vi "探头窗口-8-网络版.vi"() -> ()   [LabVIEW 2017]
panel:
  in  "外部停止命令？":bool=TRUE
  out "引用-监测模式？":refnum<vi>
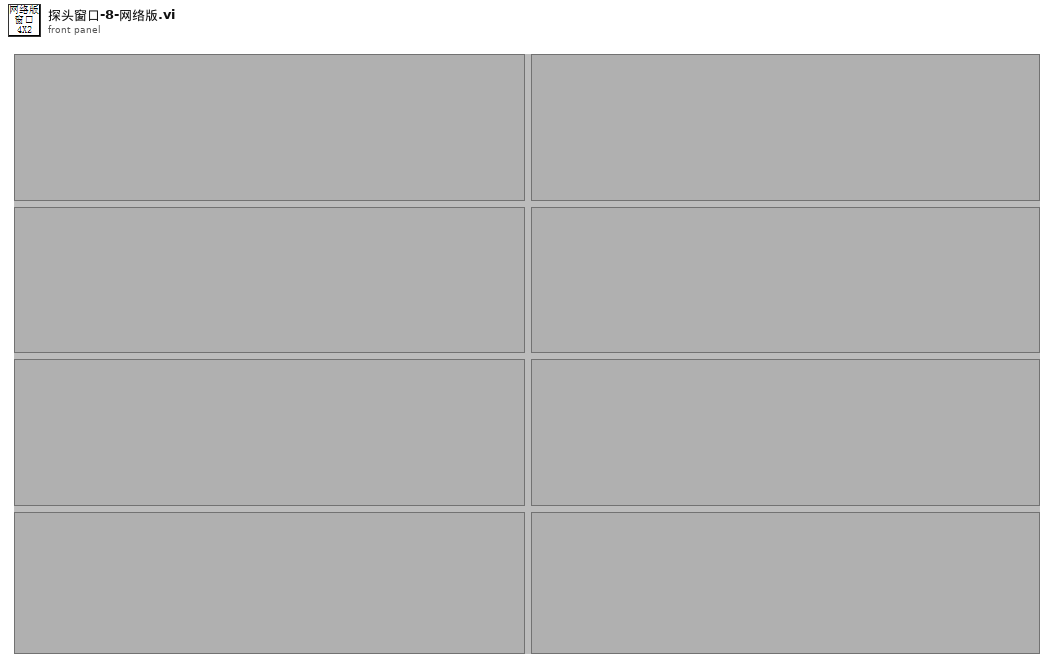
[diagram p1: front panel]
types:
  T1 = typedef "探头属性.ctl" = cluster{"探头地址与信息":T2, "测量值":T5, "限值":T6, "探头状态":T7, "累积记录":T8, "报警方式":T9}
  T2 = typedef "探测器信息.ctl" = cluster{"网络地址":string, "名称":string, "备注":string, "累积剂量":dbl, "累积限值":dbl, "硬件剂量率限值":T3, "剂量率限值1":dbl, "剂量率限值2":dbl, "报警方式":T4}
  T3 = typedef "探头剂量率限值选择.ctl" = enum16{"一级限值", "二级限值"}
  T4 = typedef "报警方式选择.ctl" = enum16{"常报警", "自动静音", "手动静音"}
  T5 = typedef "测量值.ctl" = cluster{"时间":timestamp, "数值":dbl}
  T6 = typedef "剂量率限值.ctl" = cluster{"限值1":dbl, "限值2":dbl, "探头限值":T3}
  T7 = typedef "探头状态.ctl" = enum16{"正常", "离线", "禁用", "一级报警", "二级报警", "累积报警"}
  T8 = typedef "单条累积记录.ctl" = cluster{"起始时间":timestamp, "结束时间":timestamp, "累积剂量":dbl}
  T9 = typedef "报警方式.ctl" = cluster{"报警方式":T4, "延迟计时":u16, "报警中？":bool}
  T10 = typedef "eventvkey.ctl" = enum16{"ASCII", "Enter", "Return", "Shift", "Ctrl", "Alt", "Cmd", "Opt", "Caps", "NumLock", "Clear", "Break", "Up", "Down", "Left", "Right", "Insert", "Delete", "Home", "End", "PageUp", "PageDown", "Escape", "Help", "Pause", "ScrollLock", "F1", "F2", "F3", "F4", "F5", "F6", "F7", "F8", "F9", "F10", "F11", "F12", "F13", "F14", "F15", "F16", "F17", "F18", "F19", "F20", "F21", "F22", "F23", "F24", "Play", "VolumeUp", "VolumeDown", "Mute", "Two Byte Char"}
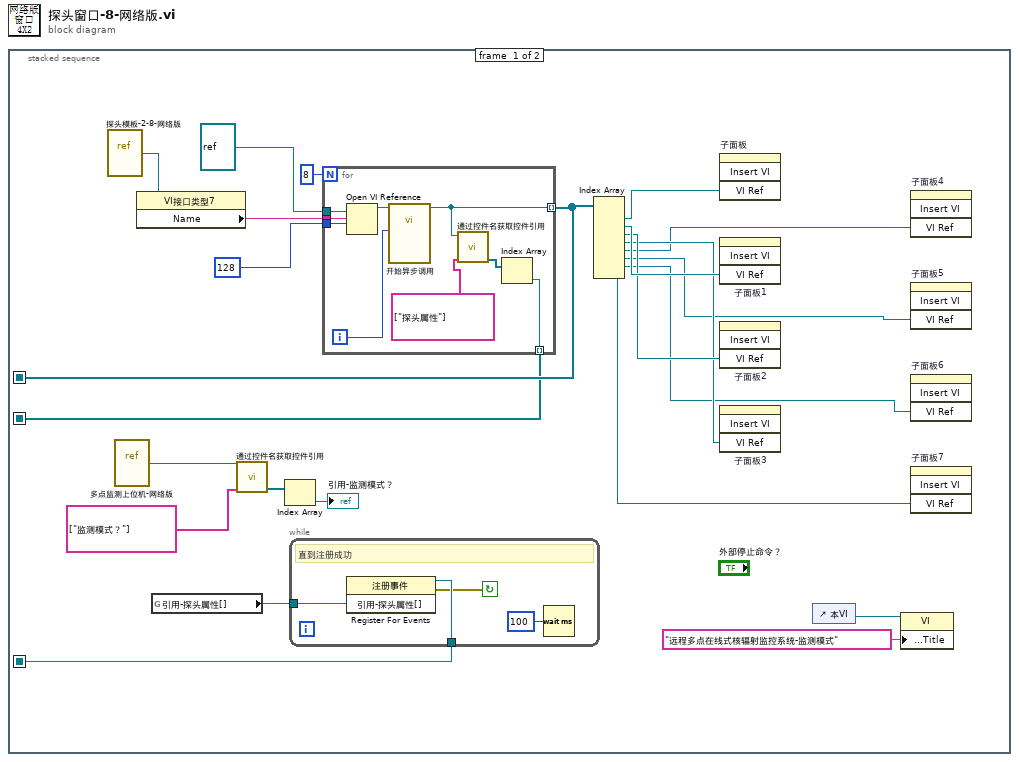
[diagram p0: block diagram]
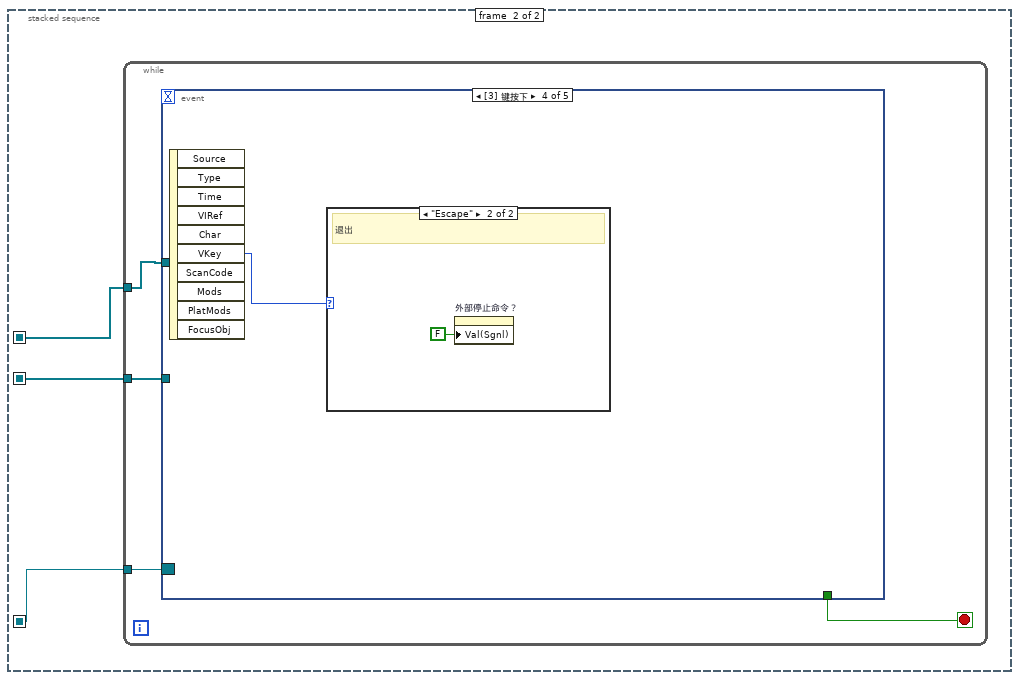
[diagram p2: hidden frame]
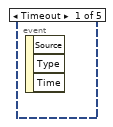
[diagram p3: hidden frame]
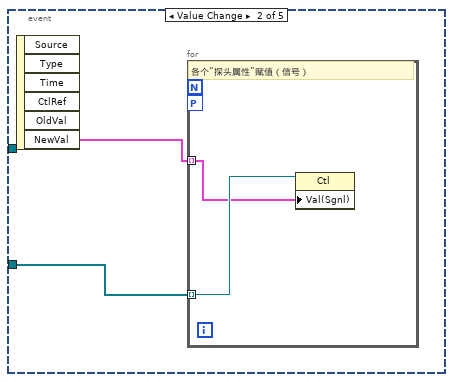
[diagram p4: hidden frame]
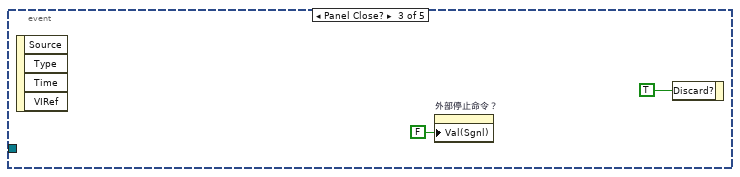
[diagram p5: hidden frame]
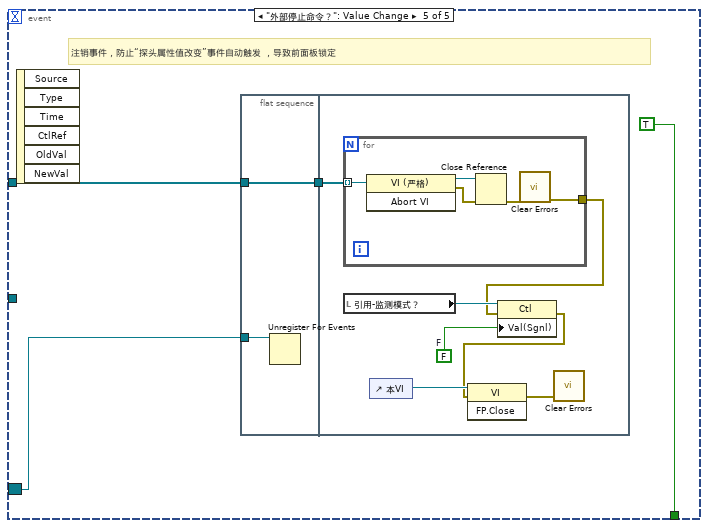
[diagram p7: hidden frame]
diagram:
  n1 = stacked-sequence {
    seq-local: [w19 _] -> [_ w39]
    seq-local: [w17 _] -> [_ w38]
    seq-local: [w1 _] -> [_ w37]
    frame #0 {
      n2 = vi-ref "探头模板-2-8-网络版.vi"() -> (w23:refnum<vi>)
      n3 = vi-ref "多点监测上位机-网络版.vi"() -> (w5:refnum<vi>)
      n4 = property class="VI接口类型7"(reference=w23) -> ("Name"=w22:string)  [unwired: 1 in, 2 out]
      n5 = global read "全局变量-35点监测.vi" "引用-探头属性[]"() -> (w2:refnum<vi>)
      n6 = call "通过控件名获取控件引用.vi"("控件名数组"=string[] ["监测模式？"], "VI引用"=w5) -> ("控件引用输出"=w7:refnum<vi>[])  [unwired: 7 in, 2 out]
      n7 = Index Array(array=w7) -> (element=→"引用-监测模式？":refnum<vi>)  [unwired: 1 in]
      n8 = while {
        tunnel: w2 -> [w27]
        tunnel: [w26] -> w1
        stop <- w25 continue-if-true
        # "直到注册成功"
        n9 = register-events(w27) -> (reference out=w26:refnum<event-registration>, error out=w25:errorcluster)  [unwired: 2 in]
        n10 = Wait (ms)(milliseconds to wait=u32 100 ("等待时间（毫秒）")) -> ()  [unwired: 1 out]
      }
      n11 = for {
        N: 8 -> [_]
        tunnel: w22 -> [w36]
        tunnel: 128 ("选项") -> [w35]
        tunnel: refnum<vi> refnum ("类型说明符VI引用句柄（仅用于类型）") -> [w34]
        tunnel: [w29] -> w19 mode=indexing
        tunnel: [w30] -> w17 mode=indexing
        i -> [w28]
        n12 = Open VI Reference(type specifier VI Refnum (for type only)=w34, vi path=w36, options=w35) -> (vi reference=w31:refnum<vi>)  [unwired: 3 in, 1 out]
        n13 = call-by-ref "开始异步调用"(reference=w31, "探头序号"=w28) -> (reference out=w29:refnum<vi>)  [unwired: 12 in, 1 out]
        n14 = call "通过控件名获取控件引用.vi"("控件名数组"=string[] ["探头属性"], "VI引用"=w29) -> ("控件引用输出"=w33:refnum<vi>[])  [unwired: 7 in, 2 out]
        n15 = Index Array(array=w33) -> (element=w30:refnum<vi>)  [unwired: 1 in]
      }
      n16 = Index Array(array=w19) -> (element #1=w16:refnum<vi>, element #2=w15:refnum<vi>, element #3=w14:refnum<vi>, element #4=w13:refnum<vi>, element #5=w12:refnum<vi>, element #6=w11:refnum<vi>, element #7=w10:refnum<vi>, element #8=w9:refnum<vi>)  [unwired: 8 in]
      n17 = invoke on="子面板" class="SubPnl" method="Insert VI"("VI Ref"=w16) -> ()  [unwired: 3 in, 4 out]
      n18 = invoke on="子面板1" class="SubPnl" method="Insert VI"("VI Ref"=w15) -> ()  [unwired: 3 in, 4 out]
      n19 = invoke on="子面板2" class="SubPnl" method="Insert VI"("VI Ref"=w14) -> ()  [unwired: 3 in, 4 out]
      n20 = invoke on="子面板3" class="SubPnl" method="Insert VI"("VI Ref"=w13) -> ()  [unwired: 3 in, 4 out]
      n21 = control-ref of="本VI"() -> (w4:refnum<vi>)
      n22 = property class="VI"(reference=w4, "Front Panel.Title"="远程多点在线式核辐射监控系统-监测模式" ("前面板窗口:标题")) -> ()  [unwired: 1 in, 2 out]
      n23 = invoke on="子面板4" class="SubPnl" method="Insert VI"("VI Ref"=w12) -> ()  [unwired: 3 in, 4 out]
      n24 = invoke on="子面板5" class="SubPnl" method="Insert VI"("VI Ref"=w11) -> ()  [unwired: 3 in, 4 out]
      n25 = invoke on="子面板6" class="SubPnl" method="Insert VI"("VI Ref"=w10) -> ()  [unwired: 3 in, 4 out]
      n26 = invoke on="子面板7" class="SubPnl" method="Insert VI"("VI Ref"=w9) -> ()  [unwired: 3 in, 4 out]
    }
    frame #1 {
      n27 = while {
        tunnel: w39 -> [w42]
        tunnel: w38 -> [w41]
        tunnel: w37 -> [w40]
        stop <- w43 stop-if-true
        n28 = event shown="[3] 键按下" {
          selector: w40 -> [_ _ _ _ w52]
          dyn-events: _ -> [_ _ _ _ _]
          timeout: _ -> [_ _ _ _ _]
          tunnel: [_ _ _ _ TRUE ("放弃？")] -> w43
          tunnel: w42 -> [_ _ _ _ w54]
          tunnel: w41 -> [_ w44 _ _ _]
          event Timeout {
            n29 = event-data() -> ()  [unwired: 1 in, 3 out]
          }
          event Value Change {
            n30 = event-data() -> ("NewVal"=w45:T1[])  [unwired: 1 in, 5 out]
            n31 = for {
              workers-P: _ -> [_]
              tunnel: w44 -> [w47] mode=indexing
              tunnel: w45 -> [w46] mode=indexing
              # "各个“探头属性”赋值（信号）"
              n32 = property class="Ctl"(reference=w47, "Val(Sgnl)"=w46) -> ()  [unwired: 1 in, 2 out]
            }
          }
          event Panel Close? {
            n33 = event-data() -> ()  [unwired: 1 in, 4 out]
            n34 = property on="外部停止命令？" class="Bool (严格)"("Val(Sgnl)"=FALSE ("值(信号)")) -> ()  [unwired: 2 in, 2 out]
            n35 = event-data("Discard?"=TRUE ("放弃？")) -> ()  [unwired: 1 in, 1 out]
          }
          event Key Down {
            n36 = event-data() -> ("VKey"=w50:T10)  [unwired: 1 in, 9 out]
            n37 = case shown="\"Escape\"" w50 {
              frame "ASCII", Default {
              }
              frame "Escape" {
                # "退出"
                n38 = property on="外部停止命令？" class="Bool (严格)"("Val(Sgnl)"=FALSE ("值(信号)")) -> ()  [unwired: 2 in, 2 out]
              }
            }
          }
          event "外部停止命令？": Value Change {
            # "注销事件，防止“探头属性值改变”事件自动触发 ，导致前面板锁定"
            n39 = event-data() -> ()  [unwired: 1 in, 6 out]
            n40 = flat-sequence {
              tunnel: w54 -> [w57]
              tunnel: [w57] -> w53
              tunnel: w52 -> [w56]
              tunnel: w53 -> [w64]
              frame #0 {
                n41 = Unregister For Events(event registration refnum=w56) -> ()  [unwired: 1 in, 1 out]
              }
              frame #1 {
                w63 = FALSE  # F
                n42 = for {
                  tunnel: w64 -> [w69] mode=indexing
                  tunnel: [w65] -> w60
                  n43 = invoke class="VI (严格)" method="Abort VI"(reference=w69) -> (reference out=w67:refnum<vi>, error out=w68:errorcluster)  [unwired: 2 in, 1 out]
                  n44 = Close Reference(reference=w67, error in (no error)=w68) -> (error out=w66:errorcluster)
                  n45 = call <vilib>:"Clear Errors.vi"("error in (no error)"=w66) -> ("error out"=w65:errorcluster)  [unwired: 5 in, 1 out]
                }
                n46 = local read "引用-监测模式？"() -> (w62:refnum<vi>)
                n47 = control-ref of="本VI"() -> (w61:refnum<vi>)
                n48 = property class="Ctl"(reference=w62, error in=w60, "Val(Sgnl)"=w63) -> (error out=w59:errorcluster)  [unwired: 1 out]
                n49 = invoke class="VI" method="FP.Close"(reference=w61, error in=w59) -> (error out=w58:errorcluster)  [unwired: 1 in, 2 out]
                n50 = call <vilib>:"Clear Errors.vi"("error in (no error)"=w58) -> ()  [unwired: 5 in, 2 out]
              }
            }
          }
        }
      }
    }
  }
